vi "GetNextProcessModule_EventRef.vi"(8 "error in (no error)":errorcluster, 9 "data":T1, 10 "source":string, 11 "Qbus in":refnum<class "Qbus.lvclass">) -> (0 "error out":errorcluster, 3 "Qbus out":refnum<class "Qbus.lvclass">)   [LabVIEW 2017, in "FileFlow.lvlib"]
doc: "Transfers an in-memory TDMS file to the message queue for the next process in the Fileflow Script. This VI looks up which process is next in order based on the value of the <B>source</B> input. If the <B>source</B> is the final process in FileflowScript, this VI sends a SendTDMSFileinMemory message to the File Manager process. File Manager manages complete files until they are transferred to the server."
uses:
  <vilib>/addons/InsightCM/Devices/Shared/Common/FileFlow/FileFlow.lvlib
  <vilib>/addons/Qbus/Qbus.lvclass
  <vilib>/addons/InsightCM/Devices/Shared/Common/FileFlow/controls/data_eventRef.ctl
  <vilib>/addons/InsightCM/Devices/Shared/Common/DataEvent/controls/EventReference.ctl
  <vilib>/addons/InsightCM/Devices/Shared/Common/DataEvent/controls/Event.ctl
  <vilib>/addons/InsightCM/MessageBus/Base/controls/DataEvent.ctl
  <vilib>/addons/InsightCM/MessageBus/Base/controls/KeyValuePair.ctl
  <vilib>/addons/InsightCM/Devices/Shared/Common/DataEvent/controls/DataSet.ctl
  <vilib>/addons/InsightCM/MessageBus/Base/controls/DataSetMetadata.ctl
  <vilib>/addons/InsightCM/MessageBus/Base/controls/TrendPoint.ctl
  <vilib>/addons/InsightCM/MessageBus/Base/controls/TrendAlarmUpdate.ctl
  <vilib>/addons/InsightCM/MessageBus/Base/controls/TrendAlarmTransition.ctl
  <vilib>/addons/PointValueMap/controls/PointMap.ctl
  <vilib>/addons/InsightCM/Devices/Shared/Common/FileManager/controls/SendEventRefRoutedMessage.ctl
  <vilib>/addons/InsightCM/Devices/Shared/Common/DataEvent/DataEvent.lvlib
  <vilib>/addons/InsightCM/Devices/Shared/Common/FileManager/FileManager.lvlib
  <vilib>/addons/PointValueMap/PointValueMap.lvlib
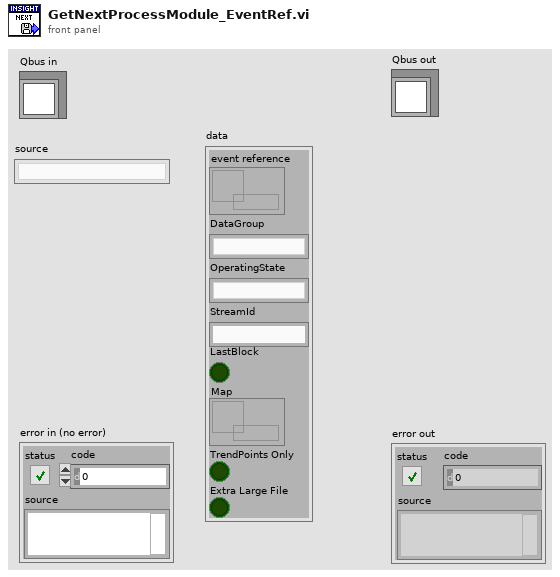
[diagram p1: front panel]
types:
  T1 = typedef "FileFlow.lvlib/data_eventRef.ctl" = cluster{"event reference":T2, "DataGroup":string, "OperatingState":string, "StreamId":string, "LastBlock":bool, "Map":T3, "TrendPoints Only":bool, "Extra Large File":bool}
  T2 = typedef "DataEvent.lvlib/EventReference.ctl" = refnum<data-value>
  T3 = typedef "PointValueMap.lvlib/PointMap.ctl" = refnum<data-value>
  T4 = typedef "FileManager.lvlib/SendEventRefRoutedMessage.ctl" = cluster{"event reference":T2, "DataGroup":string, "OperatingState":string, "StreamId":string, "LastBlock":bool, "TrendPoints Only":bool, "ExtraLargeFile":bool}
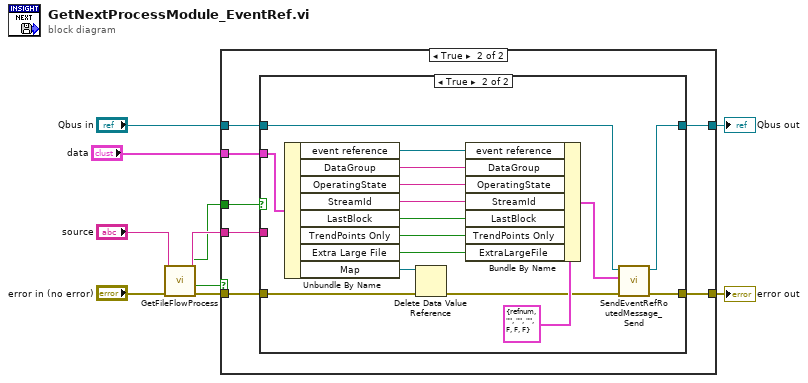
[diagram p0: block diagram]
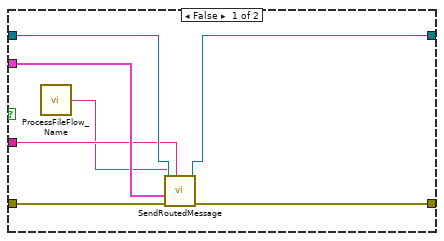
[diagram p3: hidden frame]
diagram:
  n1 = call <vilib>:"GetFileFlowProcess.vi"("error in (no error)"="error in (no error)", "source"="source") -> ("error out"=w5:errorcluster, "found"=w2:bool, "last block"=w1:bool, "Fileflow process"=w3:string)  [unwired: 6 in]
  n2 = case shown="True" w2 {
    tunnel: w5 -> [w11 w19]
    tunnel: [w11 w18] -> w10
    tunnel: [w12 w17] -> w9
    tunnel: "Qbus in" -> [w12 w16]
    tunnel: "data" -> [_ w15]
    tunnel: w3 -> [_ w14]
    tunnel: w1 -> [_ w13]
    frame False {
    }
    frame True {
      n3 = case shown="True" w13 {
        tunnel: w19 -> [w26 w41]
        tunnel: [w25 w31] -> w18
        tunnel: [w24 w33] -> w17
        tunnel: w16 -> [w23 w34]
        tunnel: w15 -> [w22 w42]
        tunnel: w14 -> [w21 _]
        frame False {
          n4 = call <vilib>:"ProcessFileFlow_Name.vi"() -> ("message name"=w20:string)  [unwired: 5 in]
          n5 = call <vilib>:"SendRoutedMessage.vi"("listener process"=w21, "error in (no error)"=w26, "message value"=w22, "message name"=w20, "Qbus in"=w23) -> ("error in (no error)"=w25:errorcluster, "Qbus out"=w24:refnum<class "Qbus.lvclass">)  [unwired: 5 in]
        }
        frame True {
          n6 = Unbundle By Name(w42) -> ("event reference"=w39:T2, "DataGroup"=w40:string, "OperatingState"=w38:string, "StreamId"=w37:string, "LastBlock"=w36:bool, "TrendPoints Only"=w29:bool, "Extra Large File"=w27:bool, "Map"=w28:T3)
          n7 = Delete Data Value Reference(data value reference=w28, error in=w41) -> (error out=w32:errorcluster)  [unwired: 1 out]
          n8 = Bundle By Name(cluster=T4 {"event reference"=refnum, "DataGroup"="", "OperatingState"="", "StreamId"="", "LastBlock"=FALSE, "TrendPoints Only"=FALSE, "ExtraLargeFile"=FALSE} ("SendEventRef"), "event reference"=w39, "DataGroup"=w40, "OperatingState"=w38, "StreamId"=w37, "LastBlock"=w36, "TrendPoints Only"=w29, "ExtraLargeFile"=w27) -> (w30:T4)
          n9 = call <vilib>:"SendEventRefRoutedMessage_Send.vi"("error in (no error)"=w32, "SendEventRef"=w30, "Qbus in"=w34) -> ("error out"=w31:errorcluster, "Qbus out"=w33:refnum<class "Qbus.lvclass">)  [unwired: 7 in]
        }
      }
    }
  }
  "error out" <- w10
  "Qbus out" <- w9
